vi "Stop Laser.vi"(8 "error in (no error)":errorcluster, 11 "Laser Process in":refnum<class "Laser Process.lvclass">) -> (0 "error out":errorcluster, 3 "Laser Process out":refnum<class "Laser Process.lvclass">)   [LabVIEW 2022 SP3, in "Laser Process.lvlib" / "Laser Process.lvclass"]
uses:
  Laser Process.lvclass
  Laser Process.lvclass/Laser Process.ctl
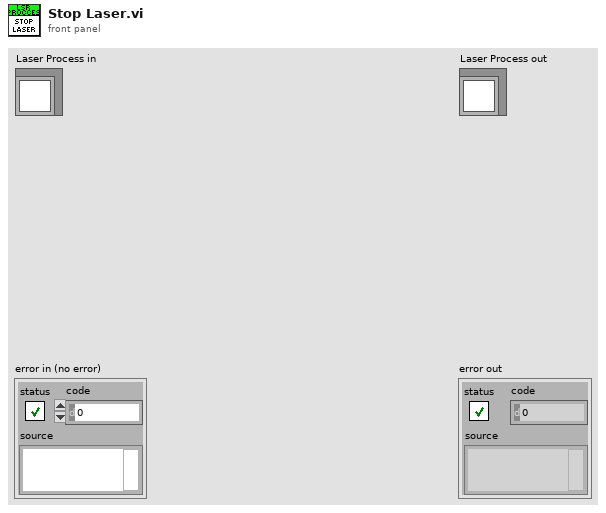
[diagram p1: front panel]
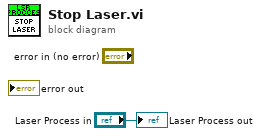
[diagram p0: block diagram]
diagram:
  "Laser Process out" <- "Laser Process in"
